vi "Tracer_Level-VI Control Data.vi"(6 "Calltree level":i32, 8 "error in (no error)":errorcluster, 9 "VI Name":string) -> (0 "error out":errorcluster, 1 "Values":string[](array[string]))   [LabVIEW 2018]
uses:
  Tracer.lvclass
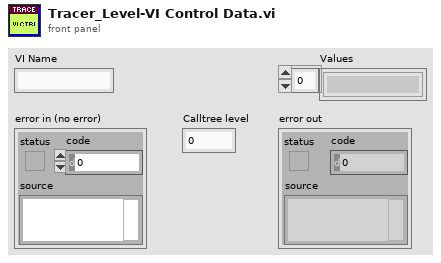
[diagram p1: front panel]
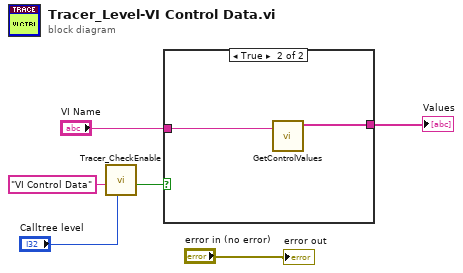
[diagram p0: block diagram]
diagram:
  n1 = call "Tracer_CheckEnable.vi"("Calltree level"="Calltree level", "Category"="VI Control Data") -> ("TraceEnabled"=w6:bool)  [unwired: 9 in]
  n2 = case shown="True" w6 {
    tunnel: "VI Name" -> [_ w8]
    tunnel: [_ w7] -> w2
    frame False {
    }
    frame True {
      n3 = call "GetControlValues.vi"("VI Name"=w8) -> ("Values"=w7:string[])  [unwired: 10 in]
    }
  }
  "Values" <- w2
  "error out" <- "error in (no error)"
